vi "Login_dialog.vi"() -> (1 "Manual mode out":bool, 2 "Experiment title out":string, 3 "User name out":string)   [LabVIEW 2011]
panel:
  in  "Login":bool
  in  "Manual mode":bool
  in  "Experiment title":string
  in  "User name":string
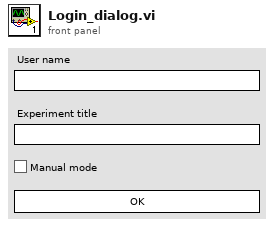
[diagram p1: front panel]
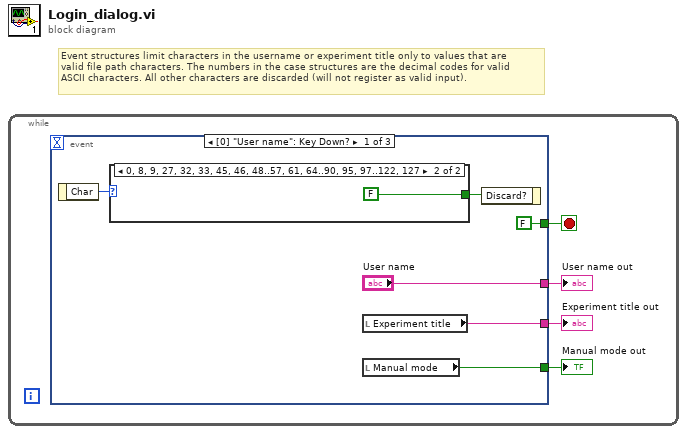
[diagram p0: block diagram]
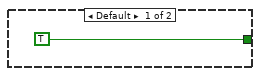
[diagram p2: hidden frame]
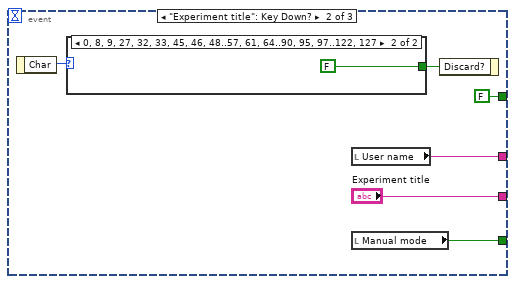
[diagram p3: hidden frame]
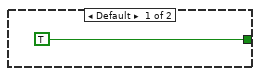
[diagram p4: hidden frame]
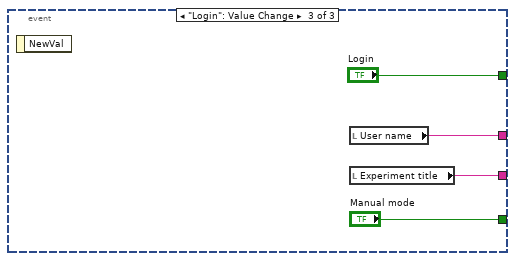
[diagram p5: hidden frame]
diagram:
  # "Event structures limit characters in the username or experiment title only to values that are\nvalid file path characters. The numbers in the case structures are the decimal codes for valid\nASCII characters. All other characters are discarded (will not register as valid input)."
  n1 = while {
    stop <- w4 stop-if-true
    n2 = event shown="[0] \"User name\": Key Down?" {
      selector: _ -> [_ _ _]
      dyn-events: _ -> [_ _ _]
      timeout: _ -> [_ _ _]
      tunnel: [FALSE ("NewVal") FALSE ("NewVal") "Login"] -> w4
      tunnel: ["User name" w15 w23] -> w3
      tunnel: [w6 "Experiment title" w22] -> w2
      tunnel: [w5 w13 "Manual mode"] -> w1
      event "User name": Key Down? {
        n3 = event-data() -> ("Char"=w10:i16)  [unwired: 1 in]
        n4 = case shown="0, 8, 9, 27, 32, 33, 45, 46, 48..57, 61, 64..90, 95, 97..122, 127" w10 {
          tunnel: [TRUE FALSE] -> w9
          frame Default {
          }
          frame 0, 8, 9, 27, 32, 33, 45, 46, 48..57, 61, 64..90, 95, 97..122, 127 {
          }
        }
        n5 = local read "Experiment title"() -> (w6:string)
        n6 = local read "Manual mode"() -> (w5:bool)
        n7 = event-data("Discard?"=w9) -> ()  [unwired: 1 in, 1 out]
      }
      event "Experiment title": Key Down? {
        n8 = event-data() -> ("Char"=w18:i16)  [unwired: 1 in]
        n9 = case shown="0, 8, 9, 27, 32, 33, 45, 46, 48..57, 61, 64..90, 95, 97..122, 127" w18 {
          tunnel: [TRUE FALSE] -> w17
          frame Default {
          }
          frame 0, 8, 9, 27, 32, 33, 45, 46, 48..57, 61, 64..90, 95, 97..122, 127 {
          }
        }
        n10 = local read "User name"() -> (w15:string)
        n11 = local read "Manual mode"() -> (w13:bool)
        n12 = event-data("Discard?"=w17) -> ()  [unwired: 1 in, 1 out]
      }
      event "Login": Value Change {
        n13 = event-data() -> ()  [unwired: 1 in, 1 out]
        n14 = local read "User name"() -> (w23:string)
        n15 = local read "Experiment title"() -> (w22:string)
      }
    }
    "User name out" <- w3
    "Experiment title out" <- w2
    "Manual mode out" <- w1
  }
